vi "VI Tree.vi"   [LabVIEW 2017, in "Roboteq Controller KBL1xxx.lvlib"]
doc: "This is the instrument driver for the <INSTRUMENT NAME>. The VI Tree displays all the user-callable VIs of the instrument driver in an organized table."
uses:
  <instrlib>/Roboteq Controller KBL1xxx/Roboteq Controller KBL1xxx.lvlib
panel:
  # "SEE DIAGRAM\nFOR VI TREE."
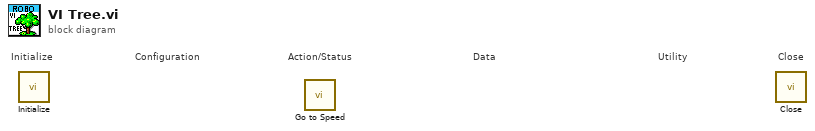
[diagram p0: block diagram]
diagram:
  # "Configuration"
  # "Utility"
  # "Data"
  # "Action/Status"
  # "Close"
  # "Initialize"
  n1 = call <instrlib>:"Initialize.vi"() -> ()  [unwired: 10 in, 2 out]
  n2 = call <instrlib>:"Go to Speed.vi"() -> ()  [unwired: 9 in, 3 out]
  n3 = call <instrlib>:"Close.vi"() -> ()  [unwired: 11 in, 1 out]
